vi "Transmission.vi"() -> ()   [LabVIEW 2016, in "transmission.lvlib"]
uses:
  Transmission/transmission.lvlib
  Low Energy End/Low energy.lvlib
  High Energy End/High energy.lvlib
  <vilib>/Instr/_visa.llb/VISA Open Access Mode.ctl
  save load/SaveLoad.lvlib
  save load/saveloadprev.ctl
panel:
  in  "Tab Control":T1(tab)
  in  "ExB Electric":dbl(slide) min=0.0 max=200.0 scale=33.0..36.0
  out "Trans Steerer Y Read":dbl format="%#.3g"
  out "Trans Steerer X Read":dbl format="%#.3g"
  in  "Transmission Y steerer":dbl(slide) min=-10.0 max=10.0 scale=-10.0..10.0
  in  "Transmission Quad A":dbl(slide) min=0.0 max=200.0 scale=5.0..120.0
  out "Switch magnet":bool=TRUE
  in  "Transmission X steerer":dbl(slide) min=-10.0 max=10.0 scale=-10.0..10.0
  out "Transmission Steerer":bool
  out "Transmission quad Range":bool
  in  "Transmission Quad B":dbl(slide) min=0.0 max=200.0 scale=6.0..120.0
  in  "stop":bool
  out "ExB":bool
  out "ExB Voltage Read-":dbl format="%#.3g"
  in  "ExB Magnet":dbl(slide) scale=0.0..10.0
  out "Switch magnet cup":bool
  out "ExB Voltage Read +":dbl format="%#.3g"
  in  "Switch magnet set":dbl(slide)=0.8365 min=0.0 max=1.6 scale=0.4..0.7
  out "Switch magnet readback":dbl(graph)=0.8365
  out "Quad A I read":string
  out "Quad A V read":string
  out "Quad B I read":string
  out "Quad B V read":string
  in  "Preview-Save-Load":T2
  in  "Trans temp file":path=path "D:/Main Tune Parameters/Temp Configs/Transmission.txt"
  in  "Quad A - VISA GPIB Resource":refnum<visa-resource-name>="GPIB2::8::INSTR"
  in  "Quad B - VISA GPIB Resource":refnum<visa-resource-name>="GPIB2::12::INSTR"
  out "ExB +READ I":dbl
  out "ExB - I":dbl
  out "Trans steer +X I":dbl
  out "Trans steer -X  I":dbl
  out "Trans steer +Y I":dbl
  out "Trans steer -Y I":dbl
  out "Trans steer +X":dbl
  out "Trans steer -X":dbl
  out "Trans steer +X Set":dbl
  out "Trans steer -X Set":dbl
  out "Trans steer +Y":dbl
  out "Trans steer -Y":dbl
  out "Trans steer +Y Set":dbl
  out "Trans steer -Y Set":dbl
  out "analyze power supply":dbl
  out "Quad B error":errorcluster
  out "Quad A error":errorcluster
  out "SaveLoad error":errorcluster
  out "SV error - event loop":errorcluster
  out "SV error - while loop":errorcluster
  # "Transmission"
  # "Quad A initially set to GPIB2::8\nQuad B initially set to GPIB2::12"
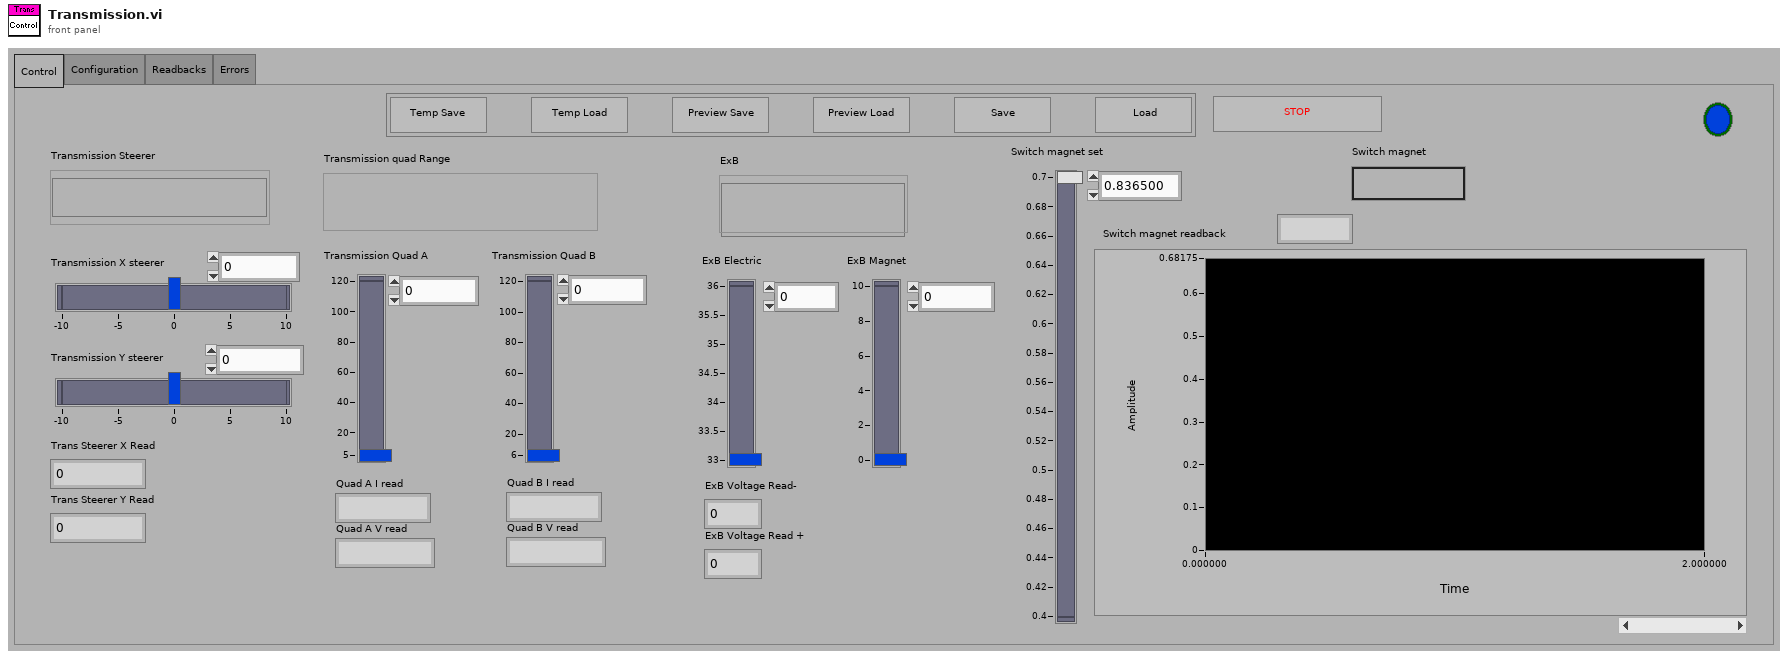
[diagram p1: front panel]
types:
  T1 = enum32{"Control", "Configuration", "Readbacks", "Errors"}
  T2 = typedef "saveloadprev.ctl" = cluster{"Temp Save":bool, "Temp Load":bool, "Save":bool, "Load":bool, "Preview Save":bool, "Preview Load":bool}
  T3 = typedef "VISA Open Access Mode.ctl" = u32
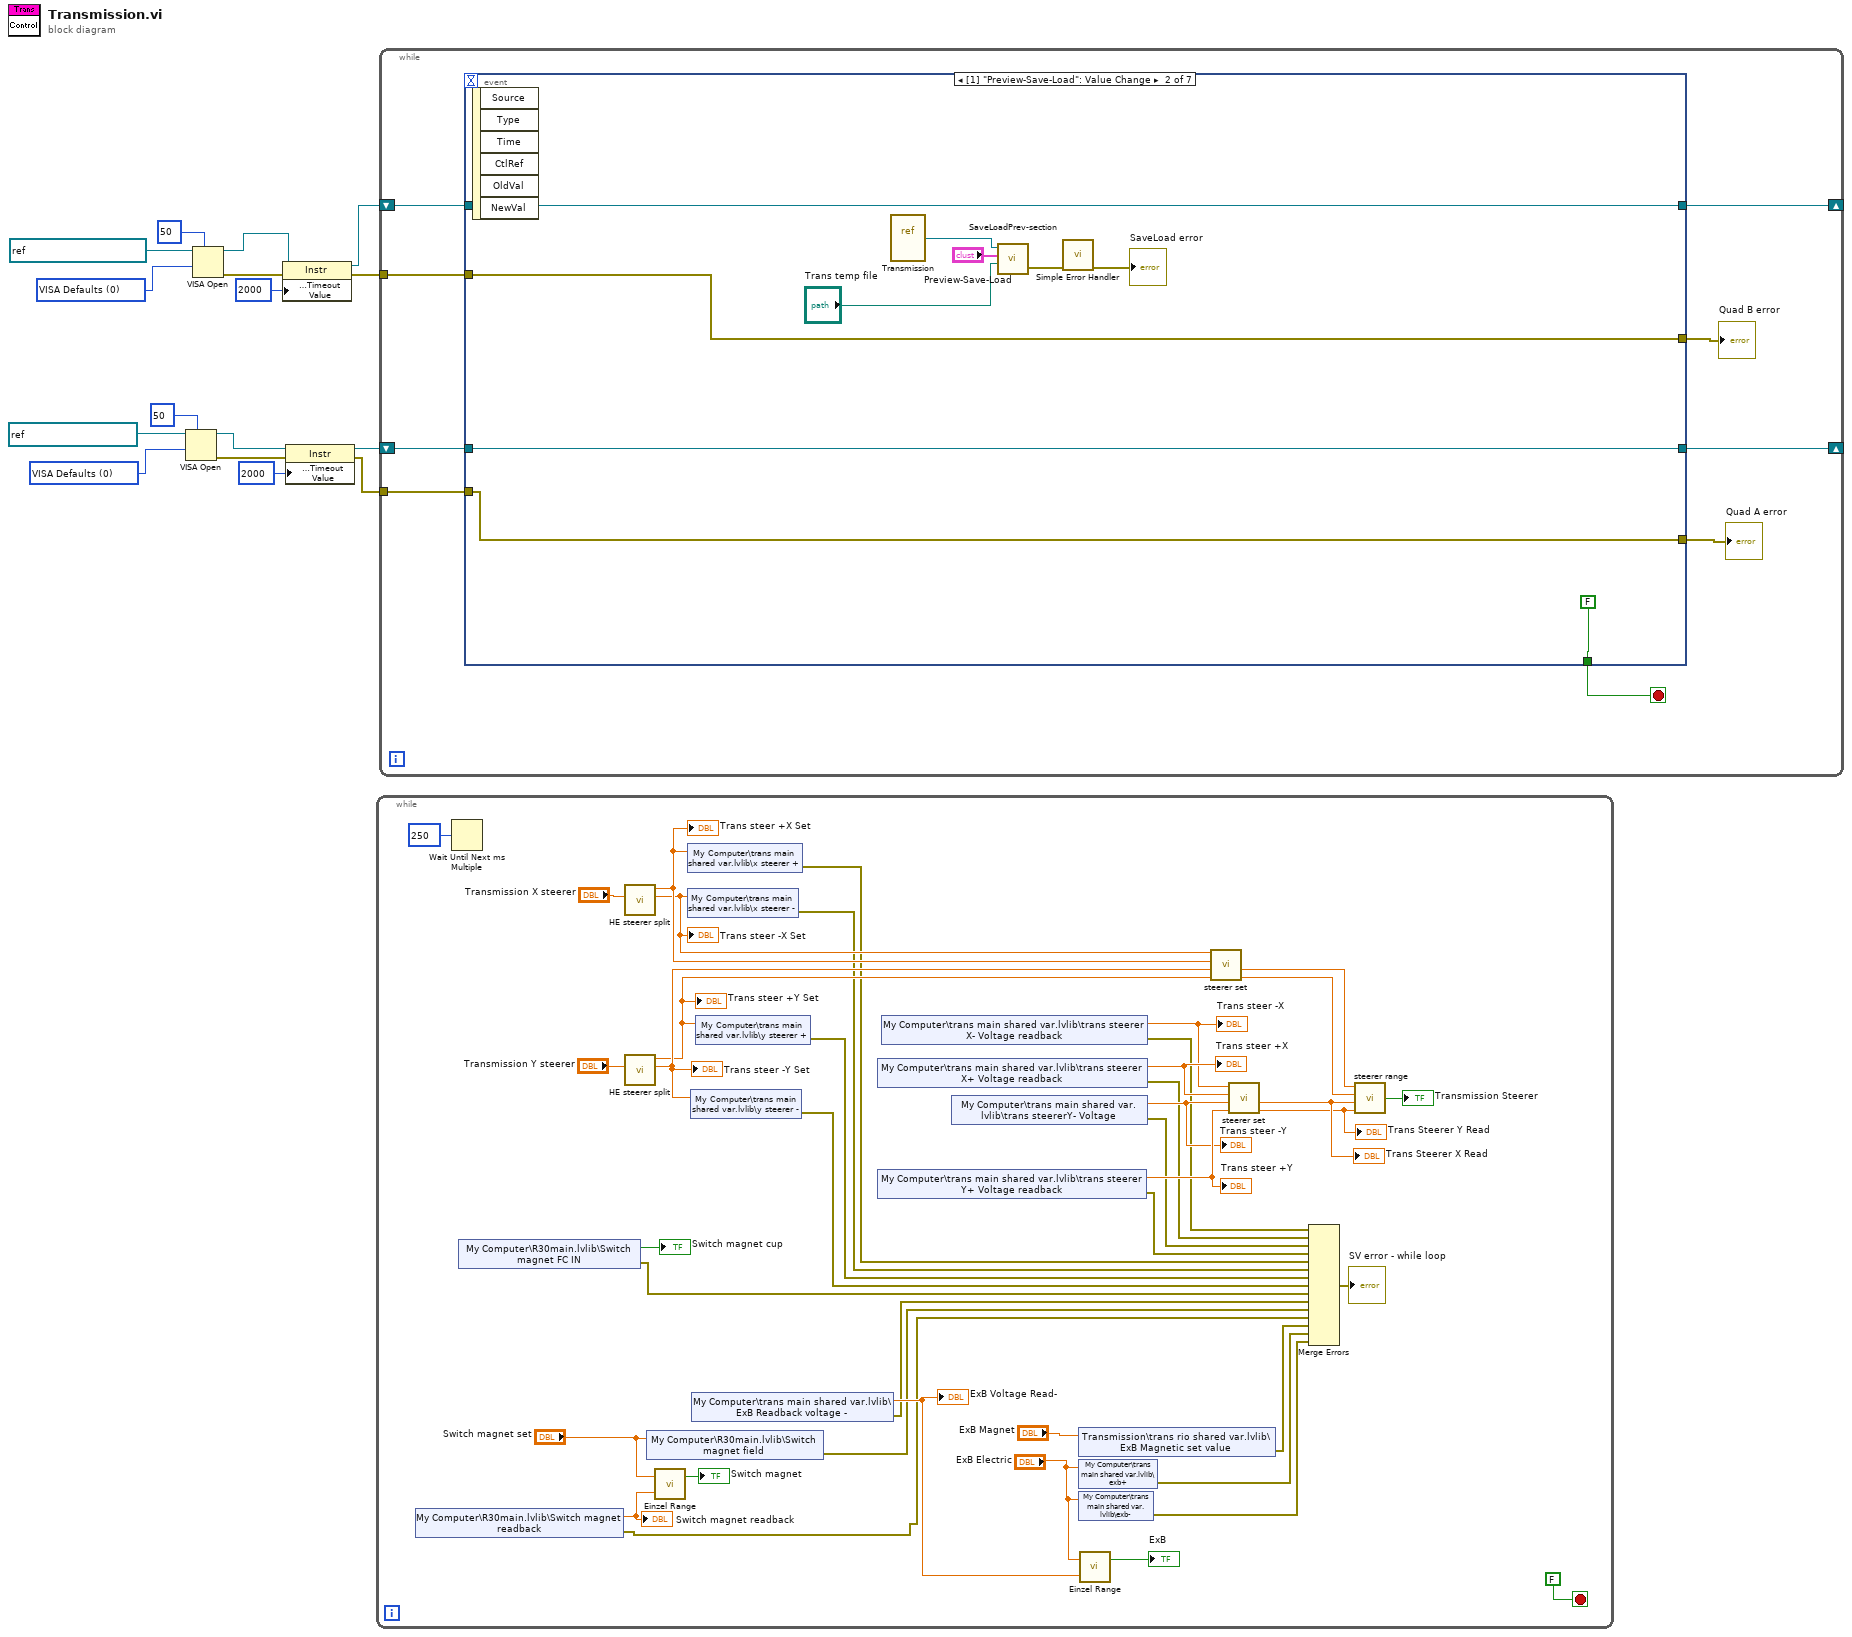
[diagram p0: block diagram]
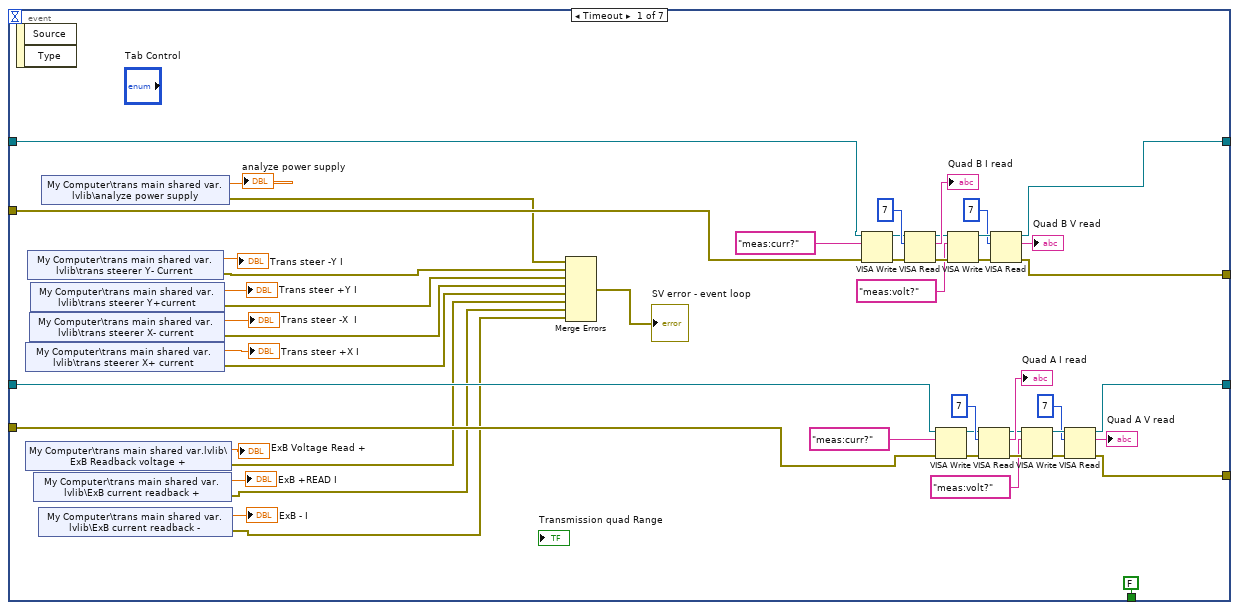
[diagram p2: hidden frame]
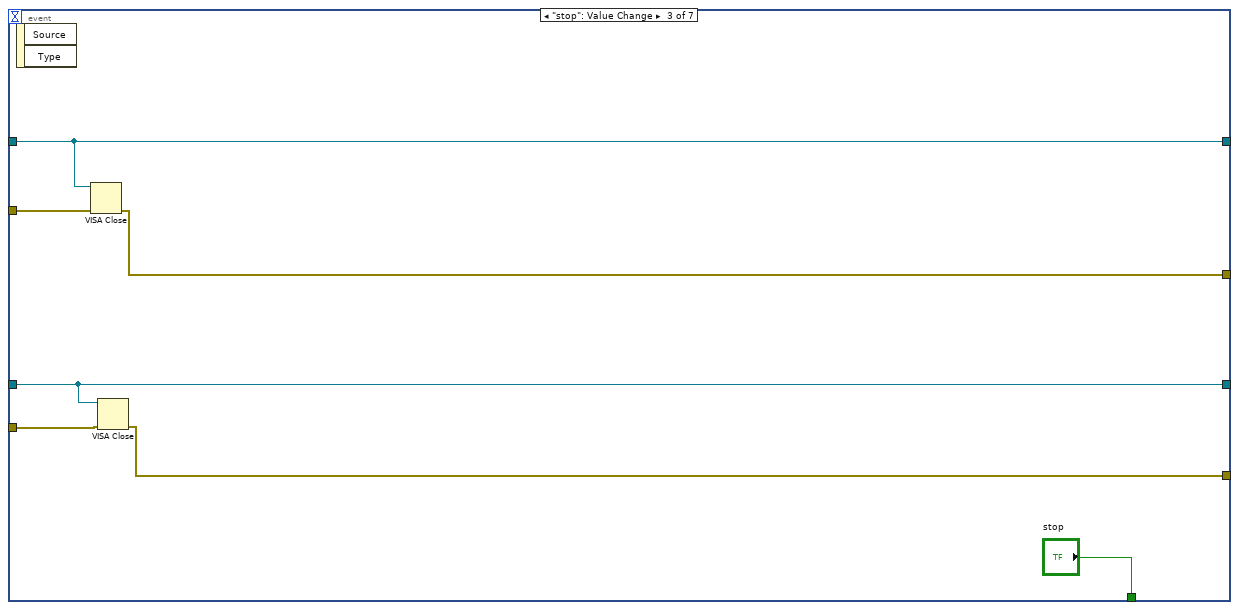
[diagram p3: hidden frame]
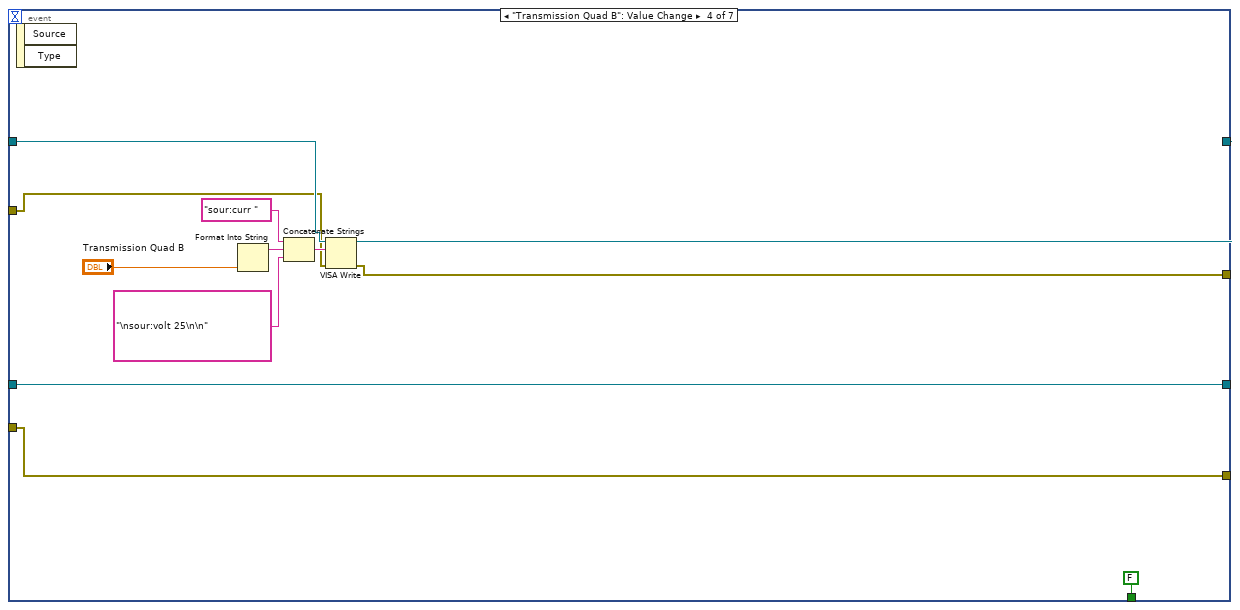
[diagram p4: hidden frame]
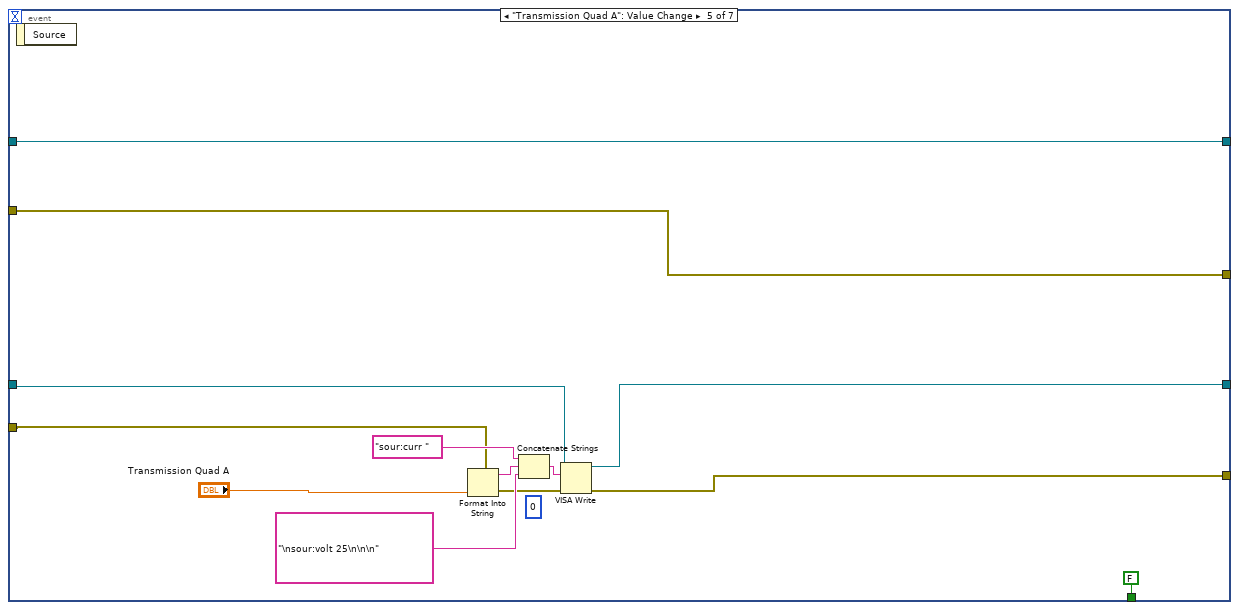
[diagram p5: hidden frame]
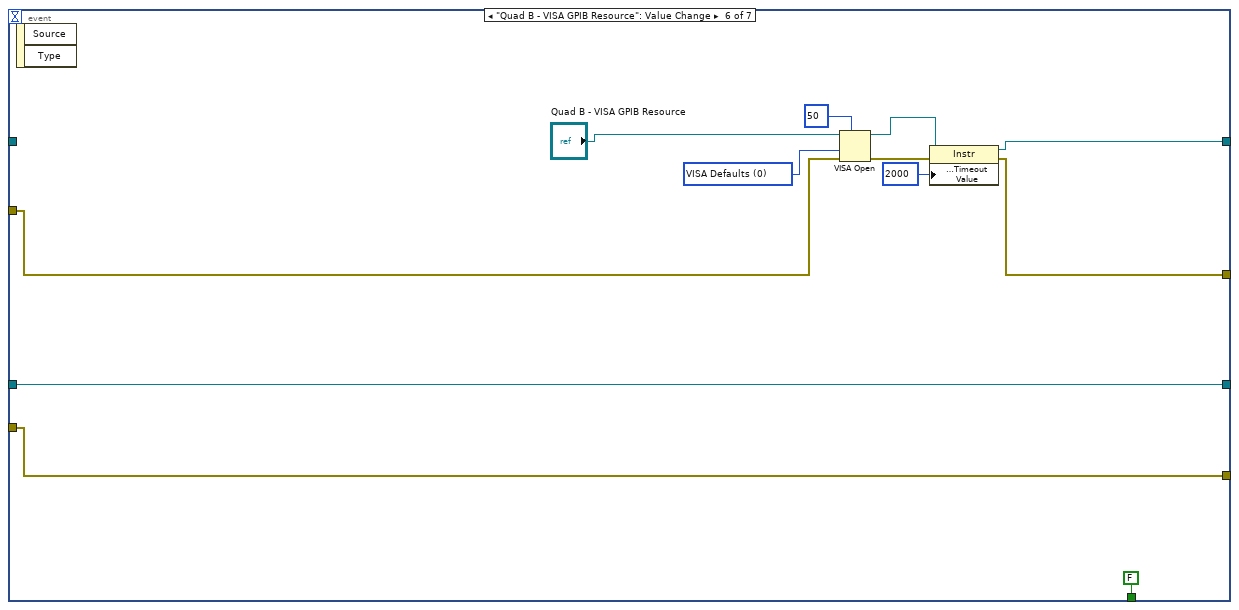
[diagram p6: hidden frame]
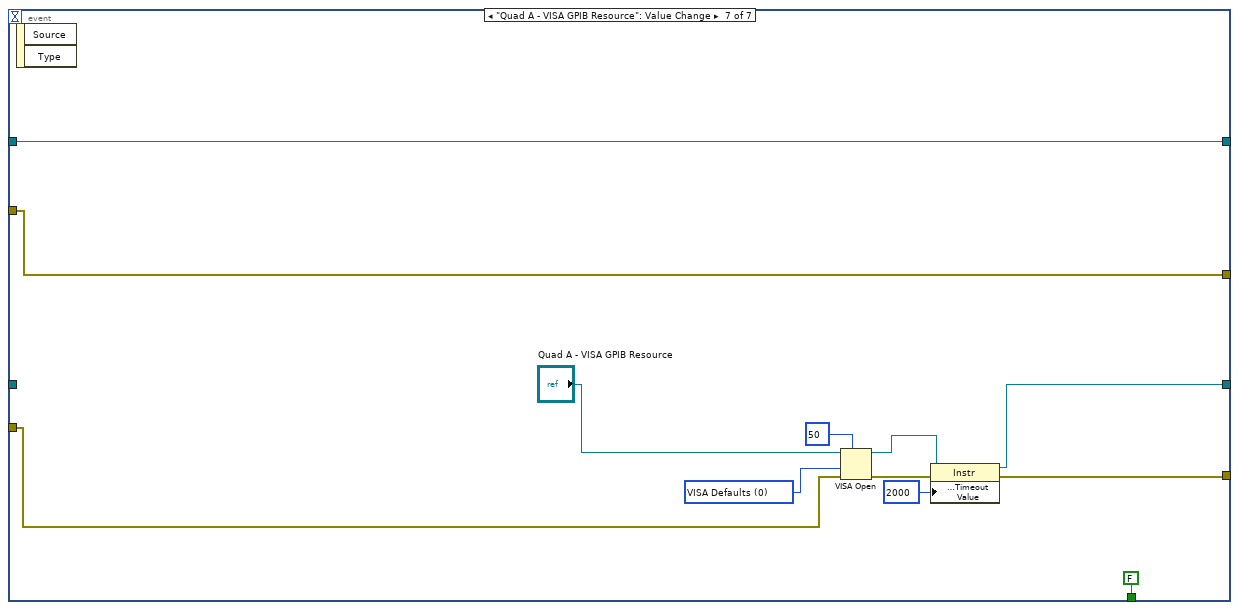
[diagram p7: hidden frame]
diagram:
  w8 = T3 0 items=["VISA Defaults"=0, "Exclusive Lock"=1, "Load Configured Settings"=4] ("Access Mode")
  w16 = T3 0 items=["VISA Defaults"=0, "Exclusive Lock"=1, "Load Configured Settings"=4] ("Access Mode")
  n1 = VISA Open(timeout (0)=u32 50 ("VISA Open timeout (0)"), access mode=w16, VISA resource name=refnum<visa-resource-name> "GPIB2::8::INSTR" ("Quad A - VISA GPIB Resource 2")) -> (VISA resource name=w13:refnum<visa-resource-name>, error out=w12:errorcluster)  [unwired: 2 in]
  n2 = VISA Open(timeout (0)=u32 50 ("VISA Open timeout (0)"), access mode=w8, VISA resource name=refnum<visa-resource-name> "GPIB2::12::INSTR" ("Quad B - VISA GPIB Resource 2")) -> (VISA resource name=w10:refnum<visa-resource-name>, error out=w11:errorcluster)  [unwired: 2 in]
  n3 = property class="Instr"(reference=w10, error in=w11, "General Settings:Timeout Value"=u32 2000) -> (reference out=w6:refnum<visa-resource-name>, error out=w5:errorcluster)
  n4 = property class="Instr"(reference=w13, error in=w12, "General Settings:Timeout Value"=u32 2000) -> (reference out=w4:refnum<visa-resource-name>, error out=w3:errorcluster)
  n5 = while {
    stop <- FALSE stop-if-true
    n6 = shared-variable "My Computer\\R30main.lvlib\\Switch magnet readback"() -> (w38:dbl, error out=w23:errorcluster)  [unwired: 1 in]
    "Switch magnet readback" <- w38
    n7 = Wait Until Next ms Multiple(millisecond multiple=u32 250) -> ()  [unwired: 1 out]
    n8 = shared-variable "My Computer\\R30main.lvlib\\Switch magnet FC IN"() -> (→"Switch magnet cup":bool, error out=w24:errorcluster)  [unwired: 1 in]
    n9 = call "HE steerer split.vi"("Steerer in"="Transmission X steerer") -> ("Steerer +"=w44:dbl, "Steerer -"=w43:dbl)  [unwired: 7 in]
    "Trans steer +X Set" <- w44
    "Trans steer -X Set" <- w43
    n10 = call "HE steerer split.vi"("Steerer in"="Transmission Y steerer") -> ("Steerer +"=w41:dbl, "Steerer -"=w42:dbl)  [unwired: 7 in]
    "Trans steer +Y Set" <- w41
    "Trans steer -Y Set" <- w42
    n11 = shared-variable "My Computer\\R30main.lvlib\\Switch magnet field"("Switch magnet set") -> (error out=w22:errorcluster)  [unwired: 1 in]
    n12 = call "Einzel Range.vi"("Inj image Readback"=w38, "Inj image Einzel Set"="Switch magnet set") -> ("Einzel  Range"=→"Switch magnet":bool)  [unwired: 1 out]
    n13 = shared-variable "My Computer\\trans main shared var.lvlib\\x steerer +"(w44) -> (error out=w28:errorcluster)  [unwired: 1 in]
    n14 = shared-variable "My Computer\\trans main shared var.lvlib\\x steerer -"(w43) -> (error out=w27:errorcluster)  [unwired: 1 in]
    n15 = shared-variable "My Computer\\trans main shared var.lvlib\\y steerer -"(w42) -> (error out=w25:errorcluster)  [unwired: 1 in]
    n16 = shared-variable "My Computer\\trans main shared var.lvlib\\ExB Readback voltage -"() -> (w37:dbl, error out=w21:errorcluster)  [unwired: 1 in]
    "ExB Voltage Read-" <- w37
    n17 = shared-variable "My Computer\\trans main shared var.lvlib\\y steerer +"(w41) -> (error out=w26:errorcluster)  [unwired: 1 in]
    n18 = shared-variable "My Computer\\trans main shared var.lvlib\\trans steerer X+ Voltage readback"() -> (w51:dbl, error out=w31:errorcluster)  [unwired: 1 in]
    "Trans steer +X" <- w51
    n19 = shared-variable "My Computer\\trans main shared var.lvlib\\trans steerer Y+ Voltage readback"() -> (w49:dbl, error out=w29:errorcluster)  [unwired: 1 in]
    "Trans steer +Y" <- w49
    n20 = shared-variable "My Computer\\trans main shared var.lvlib\\trans steerer X- Voltage readback"() -> (w50:dbl, error out=w32:errorcluster)  [unwired: 1 in]
    "Trans steer -X" <- w50
    n21 = shared-variable "My Computer\\trans main shared var.lvlib\\trans steererY- Voltage"() -> (w48:dbl, error out=w30:errorcluster)  [unwired: 1 in]
    "Trans steer -Y" <- w48
    n22 = shared-variable "Transmission\\trans rio shared var.lvlib\\ExB Magnetic set value"("ExB Magnet") -> (error out=w20:errorcluster)  [unwired: 1 in]
    n23 = shared-variable "My Computer\\trans main shared var.lvlib\\exb+"("ExB Electric") -> (error out=w19:errorcluster)  [unwired: 1 in]
    n24 = shared-variable "My Computer\\trans main shared var.lvlib\\exb-"("ExB Electric") -> (error out=w18:errorcluster)  [unwired: 1 in]
    n25 = call "Einzel Range.vi"("Inj image Readback"=w37, "Inj image Einzel Set"="ExB Electric") -> ("Einzel  Range"=→"ExB":bool)  [unwired: 1 out]
    n26 = call "steerer set.vi"("Injector image X  -"=w43, "Injector image X +"=w44, "Injector image Y  -"=w42, "Injector image Y +"=w41) -> ("Steerer X"=w55:dbl, "Steerer Y"=w54:dbl)  [unwired: 4 out]
    n27 = call "steerer set.vi"("Injector image X  -"=w50, "Injector image X +"=w51, "Injector image Y  -"=w48, "Injector image Y +"=w49) -> ("Steerer X"=w47:dbl, "Steerer Y"=w46:dbl)  [unwired: 4 out]
    "Trans Steerer X Read" <- w47
    "Trans Steerer Y Read" <- w46
    n28 = Merge Errors(w32, w31, w30, w29, w28, w27, w26, w25, w24, w21, w22, w23, w20, w19, w18) -> (→"SV error - while loop":errorcluster)
    n29 = call "steerer range.vi"("Steerer Y Voltage"=w46, "Steerer X Voltage"=w47, "Steerer Set Y"=w54, "Steerer X Set"=w55) -> ("Steerer within range"=→"Transmission Steerer":bool)  [unwired: 3 out]
  }
  n30 = while {
    tunnel: w5 -> [w64]
    tunnel: w3 -> [w62]
    shift-right: [w61] -> _
    shift-left: w6 -> [w65]
    shift-right: [w60] -> _
    shift-left: w4 -> [w63]
    stop <- w66 stop-if-true
    n31 = event shown="[1] \"Preview-Save-Load\": Value Change" {
      selector: _ -> [_ _ _ _ _ _ _]
      dyn-events: _ -> [_ _ _ _ _ _ _]
      timeout: _ -> [_ _ _ _ _ _ _]
      tunnel: [FALSE ("stop") FALSE ("stop") "stop" FALSE ("stop") FALSE ("stop") FALSE ("stop") FALSE ("stop")] -> w66
      tunnel: w65 -> [w78 w125 w130 w140 w147 _ w180]
      tunnel: w64 -> [w79 w124 w132 w139 w148 w159 w181]
      tunnel: w63 -> [w95 w123 w129 w138 w152 w168 _]
      tunnel: w62 -> [w94 w122 w131 w137 w151 w169 w170]
      tunnel: [w81 w125 w130 w136 w147 w160 w180] -> w61
      tunnel: [w96 w123 w129 w138 w149 w168 w172] -> w60
      tunnel: [w80 w124 w128 w135 w148 w158 w181] -> w59
      tunnel: [w97 w122 w127 w137 w150 w169 w171] -> w58
      event Timeout {
        n32 = event-data() -> ()  [unwired: 1 in, 2 out]
        n33 = shared-variable "My Computer\\trans main shared var.lvlib\\trans steerer X+ current"() -> (→"Trans steer +X I":dbl, error out=w71:errorcluster)  [unwired: 1 in]
        n34 = shared-variable "My Computer\\trans main shared var.lvlib\\ExB Readback voltage +"() -> (→"ExB Voltage Read +":dbl, error out=w70:errorcluster)  [unwired: 1 in]
        n35 = shared-variable "My Computer\\trans main shared var.lvlib\\trans steerer Y- Current"() -> (→"Trans steer -Y I":dbl, error out=w74:errorcluster)  [unwired: 1 in]
        n36 = shared-variable "My Computer\\trans main shared var.lvlib\\trans steerer X- current"() -> (→"Trans steer -X  I":dbl, error out=w72:errorcluster)  [unwired: 1 in]
        n37 = shared-variable "My Computer\\trans main shared var.lvlib\\trans steerer Y+current"() -> (→"Trans steer +Y I":dbl, error out=w73:errorcluster)  [unwired: 1 in]
        n38 = shared-variable "My Computer\\trans main shared var.lvlib\\ExB current readback +"() -> (→"ExB +READ I":dbl, error out=w69:errorcluster)  [unwired: 1 in]
        n39 = shared-variable "My Computer\\trans main shared var.lvlib\\ExB current readback -"() -> (→"ExB - I":dbl, error out=w68:errorcluster)  [unwired: 1 in]
        n40 = shared-variable "My Computer\\trans main shared var.lvlib\\analyze power supply"() -> (→"analyze power supply":dbl, error out=w75:errorcluster)  [unwired: 1 in]
        n41 = Merge Errors(w75, w74, w73, w72, w71, w70, w69, w68) -> (→"SV error - event loop":errorcluster)
        n42 = VISA Write(VISA resource name=w78, write buffer="meas:curr?", error in (no error)=w79) -> (VISA resource name out=w90:refnum<visa-resource-name>, error out=w91:errorcluster)  [unwired: 1 out]
        n43 = VISA Read(VISA resource name=w90, byte count=u32 7, error in (no error)=w91) -> (VISA resource name out=w86:refnum<visa-resource-name>, read buffer=→"Quad B I read":string, error out=w85:errorcluster)  [unwired: 1 out]
        n44 = VISA Write(VISA resource name=w95, write buffer="meas:curr?", error in (no error)=w94) -> (VISA resource name out=w106:refnum<visa-resource-name>, error out=w107:errorcluster)  [unwired: 1 out]
        n45 = VISA Write(VISA resource name=w86, write buffer="meas:volt?", error in (no error)=w85) -> (VISA resource name out=w88:refnum<visa-resource-name>, error out=w83:errorcluster)  [unwired: 1 out]
        n46 = VISA Read(VISA resource name=w106, byte count=u32 7, error in (no error)=w107) -> (VISA resource name out=w102:refnum<visa-resource-name>, read buffer=→"Quad A I read":string, error out=w101:errorcluster)  [unwired: 1 out]
        n47 = VISA Read(VISA resource name=w88, byte count=u32 7, error in (no error)=w83) -> (VISA resource name out=w81:refnum<visa-resource-name>, read buffer=→"Quad B V read":string, error out=w80:errorcluster)  [unwired: 1 out]
        n48 = VISA Write(VISA resource name=w102, write buffer="meas:volt?", error in (no error)=w101) -> (VISA resource name out=w104:refnum<visa-resource-name>, error out=w99:errorcluster)  [unwired: 1 out]
        n49 = VISA Read(VISA resource name=w104, byte count=u32 7, error in (no error)=w99) -> (VISA resource name out=w96:refnum<visa-resource-name>, read buffer=→"Quad A V read":string, error out=w97:errorcluster)  [unwired: 1 out]
      }
      event Value Change {
        n50 = event-data() -> ()  [unwired: 1 in, 6 out]
        n51 = vi-ref "Transmission.vi"() -> (w120:refnum<vi>)
        n52 = call "SaveLoadPrev-section.vi"("file path (use dialog)"="Trans temp file", "Cluster 2"="Preview-Save-Load", "VI Refnum"=w120) -> ("error out"=w118:errorcluster)  [unwired: 2 in]
        n53 = call <vilib>:"Simple Error Handler.vi"("error in (no error)"=w118) -> ("error out"=→"SaveLoad error":errorcluster)  [unwired: 4 in, 4 out]
      }
      event "stop": Value Change {
        n54 = event-data() -> ()  [unwired: 1 in, 2 out]
        n55 = VISA Close(VISA resource name=w130, error in (no error)=w132) -> (error out=w128:errorcluster)
        n56 = VISA Close(VISA resource name=w129, error in (no error)=w131) -> (error out=w127:errorcluster)
      }
      event "Transmission Quad B": Value Change {
        n57 = event-data() -> ()  [unwired: 1 in, 2 out]
        n58 = Format Into String("Transmission Quad B") -> (resulting string=w143:string)  [unwired: 3 in, 1 out]
        n59 = Concatenate Strings("sour:curr " ("string"), w143, "\nsour:volt 25\n\n" ("write buffer")) -> (w142:string)
        n60 = VISA Write(VISA resource name=w140, write buffer=w142, error in (no error)=w139) -> (VISA resource name out=w136:refnum<visa-resource-name>, error out=w135:errorcluster)  [unwired: 1 out]
      }
      event "Transmission Quad A": Value Change {
        (unwired) i16 0 ("mode (0)")
        n61 = event-data() -> ()  [unwired: 1 in, 1 out]
        n62 = Format Into String("Transmission Quad A") -> (resulting string=w154:string)  [unwired: 3 in, 1 out]
        n63 = Concatenate Strings("sour:curr " ("string"), w154, "\nsour:volt 25\n\n\n" ("write buffer")) -> (w156:string)
        n64 = VISA Write(VISA resource name=w152, write buffer=w156, error in (no error)=w151) -> (VISA resource name out=w149:refnum<visa-resource-name>, error out=w150:errorcluster)  [unwired: 1 out]
      }
      event "Quad B - VISA GPIB Resource": Value Change {
        w163 = T3 0 items=["VISA Defaults"=0, "Exclusive Lock"=1, "Load Configured Settings"=4] ("Access Mode")
        n65 = event-data() -> ()  [unwired: 1 in, 2 out]
        n66 = VISA Open(timeout (0)=u32 50 ("VISA Open timeout (0)"), access mode=w163, error in (no error)=w159, VISA resource name="Quad B - VISA GPIB Resource") -> (VISA resource name=w165:refnum<visa-resource-name>, error out=w166:errorcluster)  [unwired: 1 in]
        n67 = property class="Instr"(reference=w165, error in=w166, "General Settings:Timeout Value"=u32 2000) -> (reference out=w160:refnum<visa-resource-name>, error out=w158:errorcluster)
      }
      event "Quad A - VISA GPIB Resource": Value Change {
        w175 = T3 0 items=["VISA Defaults"=0, "Exclusive Lock"=1, "Load Configured Settings"=4] ("Access Mode")
        n68 = event-data() -> ()  [unwired: 1 in, 2 out]
        n69 = VISA Open(timeout (0)=u32 50 ("VISA Open timeout (0)"), access mode=w175, error in (no error)=w170, VISA resource name="Quad A - VISA GPIB Resource") -> (VISA resource name=w177:refnum<visa-resource-name>, error out=w178:errorcluster)  [unwired: 1 in]
        n70 = property class="Instr"(reference=w177, error in=w178, "General Settings:Timeout Value"=u32 2000) -> (reference out=w172:refnum<visa-resource-name>, error out=w171:errorcluster)
      }
    }
    "Quad B error" <- w59
    "Quad A error" <- w58
  }
